vi "Construct.vi"(8 "error in (no error)":errorcluster, 11 "SolutionBuilder in":refnum<class "SolutionBuilder.lvclass">) -> (0 "error out":errorcluster, 3 "SolutionBuilder out":refnum<class "SolutionBuilder.lvclass">)   [LabVIEW 2020, in "SolutionBuilder.lvlib" / "SolutionBuilder.lvclass"]
uses:
  SolutionBuilder.lvclass
  SolutionBuilder.lvclass/SolutionBuilder.ctl
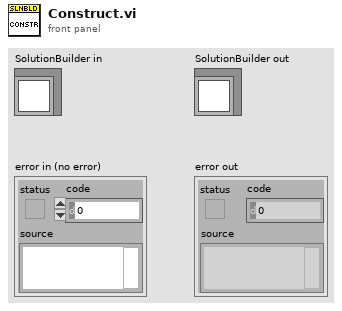
[diagram p1: front panel]
types:
  T1 = typedef "SolutionBuilder.lvlib/SolutionBuilder.lvclass/Options.ctl" = cluster{"Path":path, "Preview?":bool, "Quiet?":bool, "Log file":path, "Success file":path}
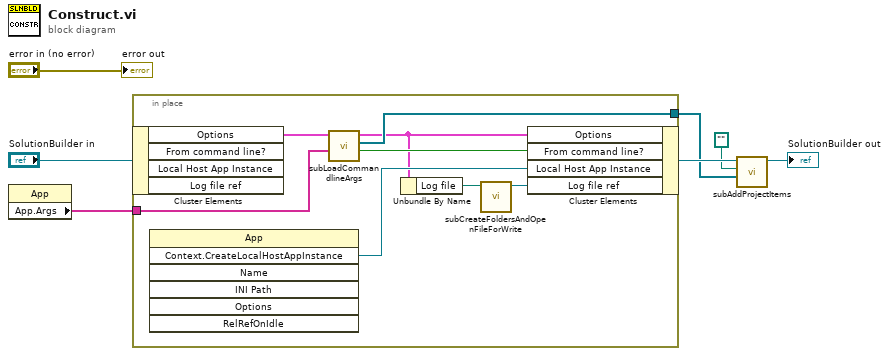
[diagram p0: block diagram]
diagram:
  n1 = property class="App"() -> ("App.Args"=w2:string[])  [unwired: 2 in, 2 out]
  n2 = in-place {
    in-place-border: [w12] -> w3
    in-place-border: w2 -> [w11]
    n3 = in-place-cluster #1("SolutionBuilder in") -> ("Options"=w15:T1)  [unwired: 3 out]
    n4 = invoke class="App" method="Context.CreateLocalHostAppInstance"() -> ("Create Context"=w13:refnum<vi>)  [unwired: 7 in, 6 out]
    n5 = call "subLoadCommandlineArgs.vi"("App.Args"=w11, "Options in"=w15) -> ("From command line?"=w14:bool, "Pre-built libraries"=w12:refnum<class "ProjectItem.lvclass">[], "Options"=w10:T1)  [unwired: 6 in, 1 out]
    n6 = Unbundle By Name(w10) -> ("Log file"=w8:path)
    n7 = call "subCreateFoldersAndOpenFileForWrite.vi"("File path"=w8) -> ("File ref"=w9:refnum<file>)  [unwired: 10 in]
    n8 = in-place-cluster #1("Options"=w10, "From command line?"=w14, "Local Host App Instance"=w13, "Log file ref"=w9) -> (w5:refnum<class "SolutionBuilder.lvclass">)
  }
  n9 = call "subAddProjectItems.vi"("ProjectItems"=w3, "Owning project"=path "", "SolutionBuilder in"=w5) -> ("SolutionBuilder out"=→"SolutionBuilder out":refnum<class "SolutionBuilder.lvclass">)  [unwired: 7 in, 1 out]
  "error out" <- "error in (no error)"
